vi "Correct_Disconnection_101_and_11_Point-1.vi"(4 "error IN":errorcluster, 7 "[IN] Still connected\ntracks in group":T2) -> (0 "error OUT":errorcluster, 3 "[OUT] Clusters for Re\nconstructed Tracks":T1)   [LabVIEW 2013]
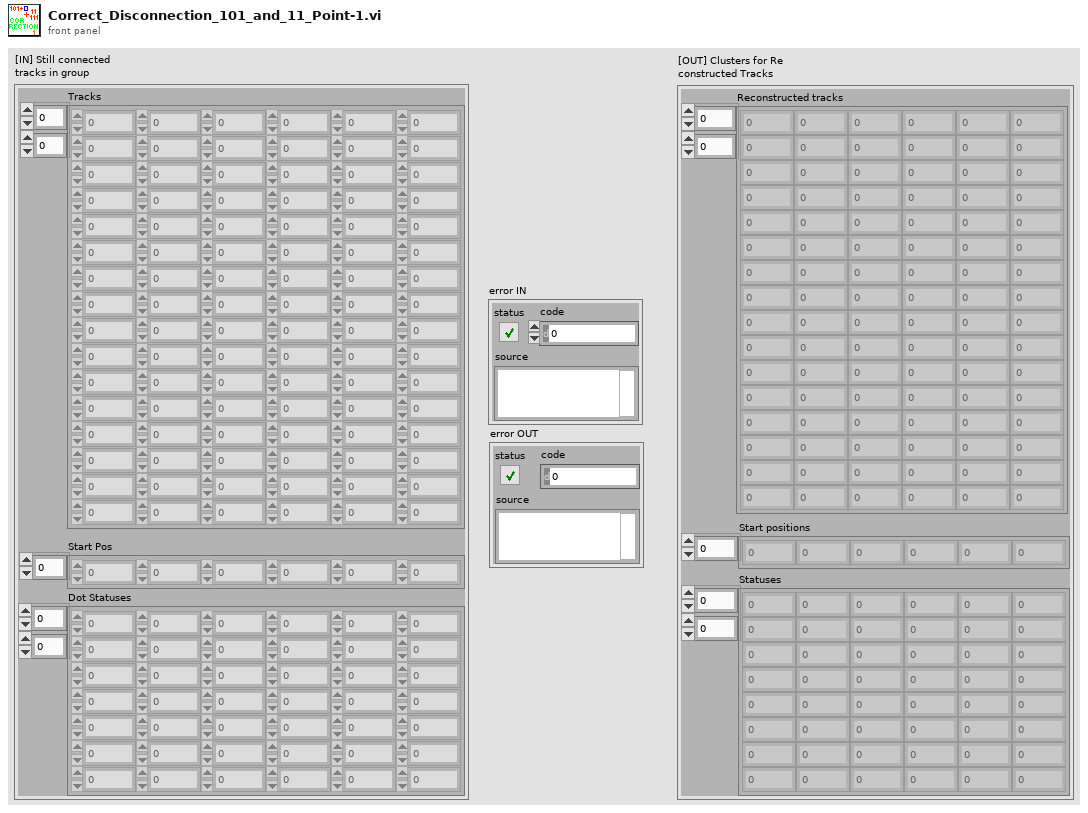
[diagram p1: front panel]
types:
  T1 = cluster{"Reconstructed tracks":dbl[][], "Start positions":i32[], "Statuses":i16[][]}
  T2 = cluster{"Tracks":dbl[][], "Start Pos":i32[], "Dot Statuses":i16[][]}
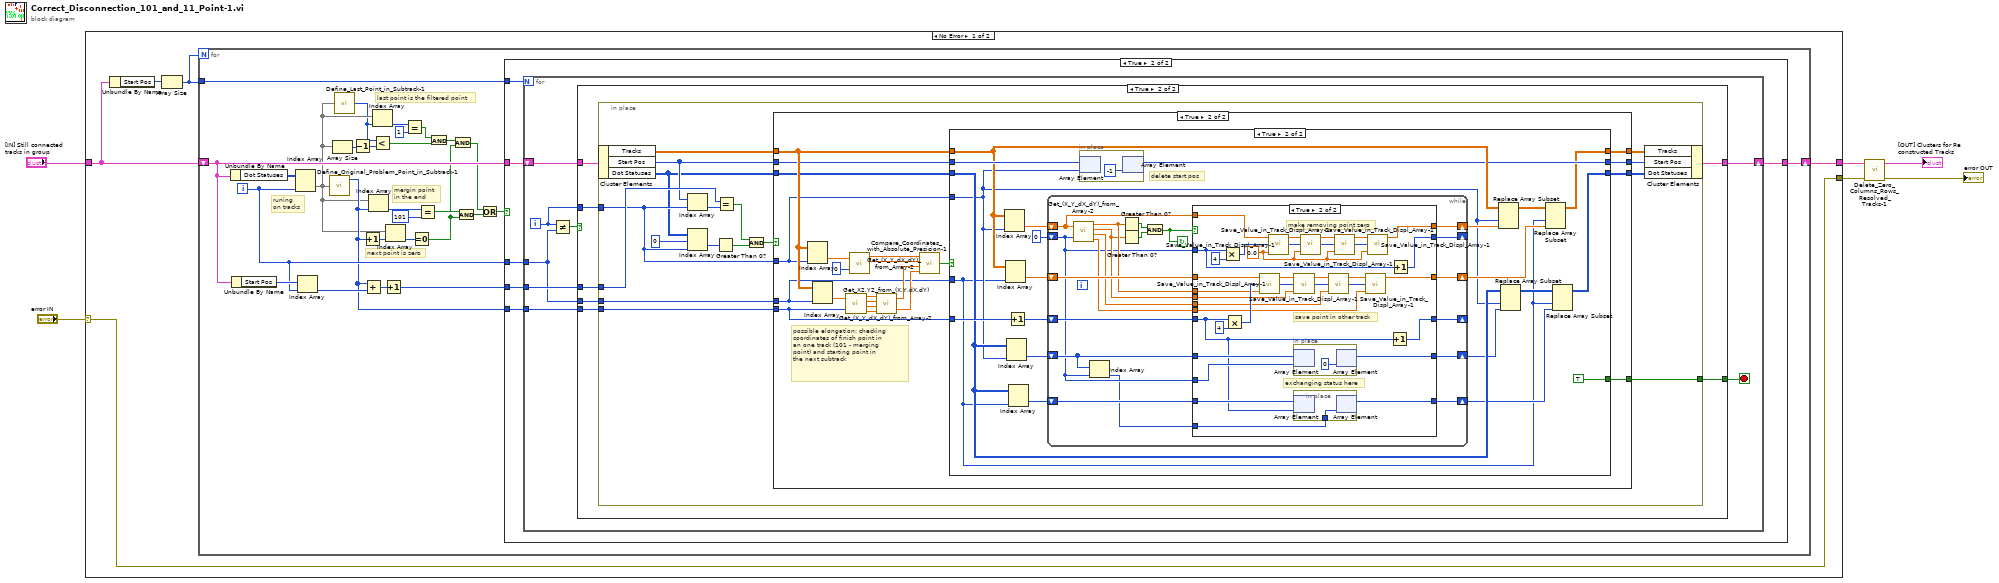
[diagram p0: block diagram]
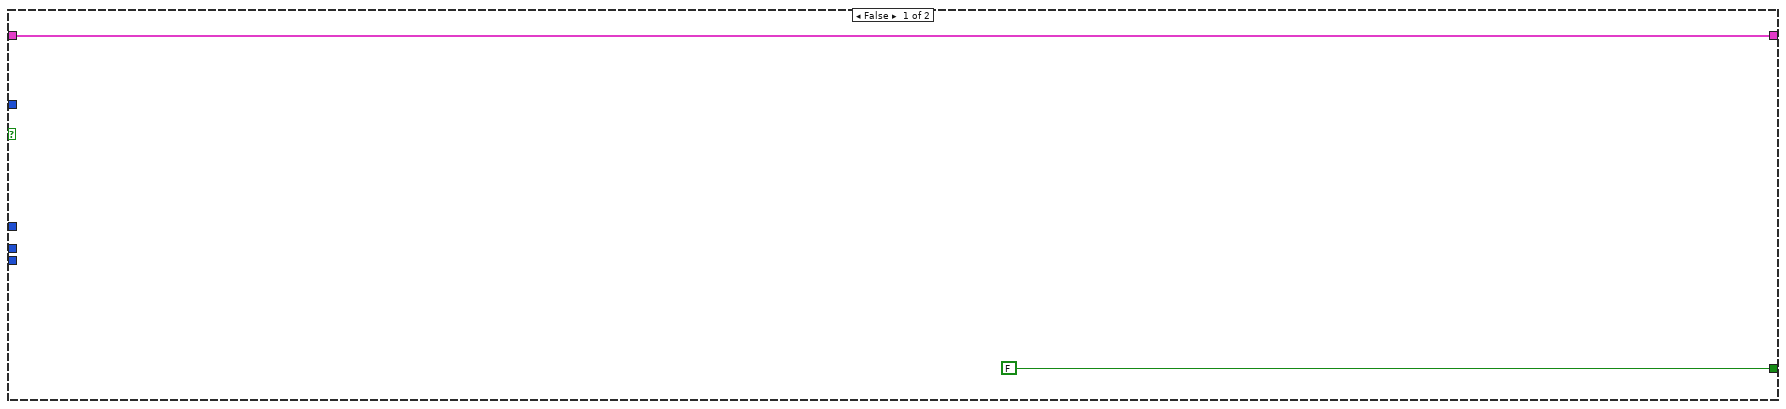
[diagram p3: hidden frame]
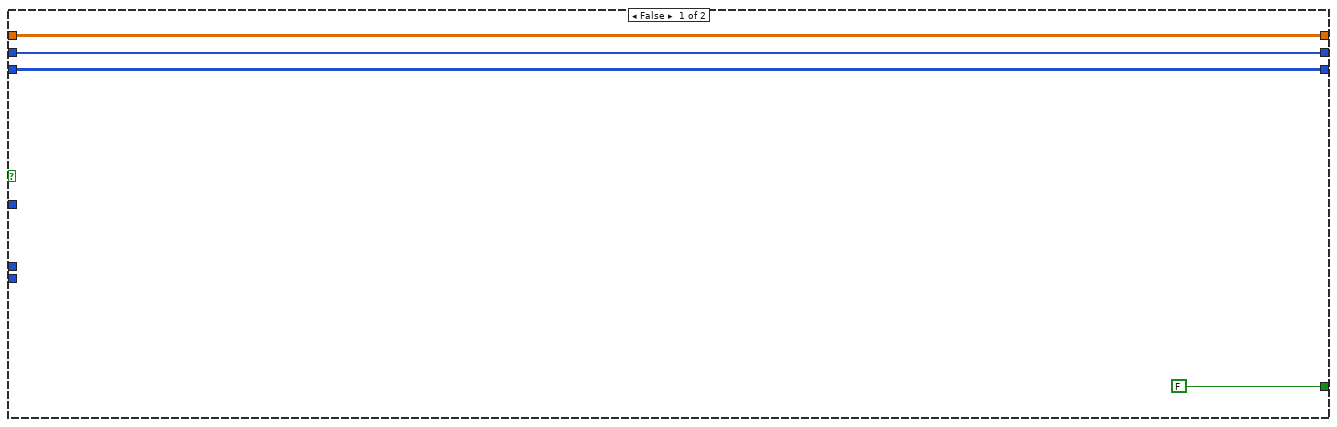
[diagram p4: hidden frame]
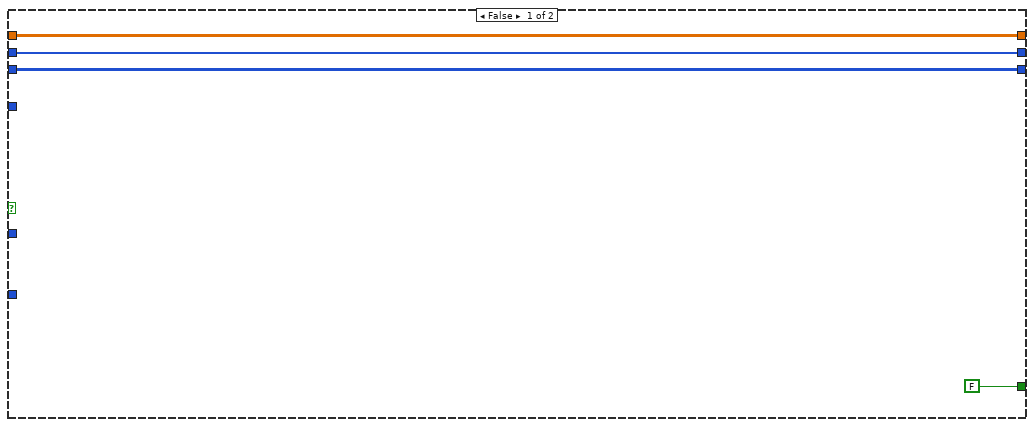
[diagram p5: hidden frame]
diagram:
  n1 = case shown="No Error" "error IN" {
    selector: "error IN" -> [w8 w197]
    tunnel: "[IN] Still connected\ntracks in group" -> [w10 w198]
    tunnel: [w8 w197] -> w3
    tunnel: [w7 w198] -> w4
    frame No Error {
      n2 = Unbundle By Name(w10) -> ("Start Pos"=w11:i32[])
      n3 = Array Size(array=w11) -> (size(s)=w9:i32)
      n4 = for {
        N: w9 -> [_]
        shift-right: [w27] -> w7
        shift-left: w10 -> [w34]
        tunnel: w9 -> [w39]
        i -> [w32]
        # "last point is the filtered point"
        # "mergin point \nin the end"
        # "runing \non tracks"
        # "next point is zero"
        n5 = Unbundle By Name(w34) -> ("Dot Statuses"=w35:i16[][])
        n6 = Unbundle By Name(w34) -> ("Start Pos"=w33:i32[])
        n7 = Index Array(array=w35, index (col)=w32) -> (element=w23:i16[])  [unwired: 1 in]
        n8 = Index Array(array=w33, index=w32) -> (element=w31:i32)
        n9 = call "Define_Original_Problem_Point_in_Subtrack-1.vi"("[IN] Statuses"=w23) -> ("[OUT] Index of Problem Point\nin Subtrack (Original)"=w28:i32)  [unwired: 3 in, 1 out]
        n10 = Array Size(array=w23) -> (size(s)=w22:i32)
        n11 = call "Define_Last_Point_in_Subtrack-1.vi"("[IN] Statuses"=w23) -> ("[OUT] Index of Problem Point\nin Subtrack (Original)"=w20:i32)  [unwired: 4 in]
        n12 = Decrement(x=w22) -> (x-1=w19:i32)
        n13 = Increment(x=w28) -> (x+1=w37:i32)
        n14 = Add(x=w28, y=w31) -> (x+y=w30:i32)
        n15 = Index Array(array=w23, index=w28) -> (element=w26:i16)
        n16 = Index Array(array=w23, index=w20) -> (element=w25:i16)
        n17 = Less?(x=w20, y=w19) -> (x < y?=w17:bool)
        n18 = Increment(x=w30) -> (x+1=w29:i32)
        n19 = Index Array(array=w23, index=w37) -> (element=w38:i16)
        n20 = Equal?(x=w25, y=i16 1) -> (x = y?=w18:bool)
        n21 = Equal To 0?(x=w38) -> (x = 0?=w15:bool)
        n22 = Equal?(x=w26, y=i16 101) -> (x = y?=w21:bool)
        n23 = And(x=w18, y=w17) -> (x .and. y?=w16:bool)
        n24 = And(x=w16, y=w15) -> (x .and. y?=w12:bool)
        n25 = And(x=w21, y=w15) -> (x .and. y?=w14:bool)
        n26 = Or(x=w12, y=w14) -> (x .or. y?=w13:bool)
        n27 = case shown="True" w13 {
          tunnel: w39 -> [_ w46]
          tunnel: w34 -> [w40 w45]
          tunnel: w32 -> [_ w44]
          tunnel: w29 -> [_ w43]
          tunnel: w28 -> [_ w42]
          tunnel: [w40 w41] -> w27
          frame False {
          }
          frame True {
            n28 = for {
              N: w46 -> [_]
              shift-right: [w48] -> w41
              shift-left: w45 -> [w53]
              tunnel: w44 -> [w50]
              tunnel: w43 -> [w51]
              tunnel: w42 -> [w49]
              i -> [w52]
              stop <- w47 stop-if-true
              n29 = Not Equal?(x=w52, y=w50) -> (x != y?=w54:bool)
              n30 = case shown="True" w54 {
                tunnel: w53 -> [w56 w63]
                tunnel: w52 -> [_ w62]
                tunnel: w51 -> [_ w61]
                tunnel: w50 -> [_ w60]
                tunnel: w49 -> [_ w59]
                tunnel: [w56 w58] -> w48
                tunnel: [FALSE w57] -> w47
                frame False {
                }
                frame True {
                  n31 = in-place {
                    in-place-border: w62 -> [w73]
                    in-place-border: w61 -> [w76]
                    in-place-border: w60 -> [w72]
                    in-place-border: w59 -> [w71]
                    in-place-border: [w65] -> w57
                    n32 = in-place-cluster #1(w63) -> ("Tracks"=w74:dbl[][], "Start Pos"=w70:i32[], "Dot Statuses"=w69:i16[][])
                    n33 = Index Array(array=w70, index=w73) -> (element=w77:i32)
                    n34 = Index Array(array=w69, index (row)=0 ("disabled index (row)"), index (col)=w73) -> (element=w78:i16)
                    n35 = Greater Than 0?(x=w78) -> (x > 0?=w64:bool)
                    n36 = Equal?(x=w76, y=w77) -> (x = y?=w79:bool)
                    n37 = And(x=w79, y=w64) -> (x .and. y?=w75:bool)
                    n38 = case shown="True" w75 {
                      tunnel: w74 -> [w84 w94]
                      tunnel: w73 -> [_ w90]
                      tunnel: w72 -> [_ w89]
                      tunnel: w71 -> [_ w91]
                      tunnel: w70 -> [w83 w93]
                      tunnel: w69 -> [w82 w92]
                      tunnel: [w83 w88] -> w68
                      tunnel: [w84 w87] -> w67
                      tunnel: [w82 w86] -> w66
                      tunnel: [FALSE w85] -> w65
                      frame False {
                      }
                      frame True {
                        # "possible elongation: checking \ncoordinates of finish point in \nan one track (101 - merging\npoint) and starting point in \nthe next subtrack"
                        n39 = Index Array(array=w94, index (col)=w90) -> (element=w106:dbl[])  [unwired: 1 in]
                        n40 = Index Array(array=w94, index (col)=w89) -> (element=w104:dbl[])  [unwired: 1 in]
                        n41 = call "Get_(X_Y_dX_dY)_from_Array-2.vi"("(X,Y,dX,dY)"=w104, "Index of Displacement"=w91) -> ("X"=w103:dbl, "Y"=w102:dbl, "dX"=w101:dbl, "dY"=w100:dbl)
                        n42 = call "Get_(X_Y_dX_dY)_from_Array-2.vi"("(X,Y,dX,dY)"=w106, "Index of Displacement"=0 ("disabled index (row)")) -> ("X"=w99:dbl, "Y"=w98:dbl)  [unwired: 2 out]
                        n43 = call "Get_X2,Y2_from_(X,Y,dX,dY).vi"("dY"=w100, "dX"=w101, "Y1"=w102, "X1"=w103) -> ("Y2 = (Y1+dY)"=w96:dbl, "X2 = (X1+dX)"=w97:dbl)
                        n44 = call "Compare_Coordinates_with_Absolute_Presicion-1.vi"("X 1"=w99, "Y 1"=w98, "X 2"=w97, "Y 2"=w96) -> ("[OUT] Same coordinates?"=w95:bool)  [unwired: 1 in]
                        n45 = case shown="True" w95 {
                          tunnel: w94 -> [w110 w124]
                          tunnel: w93 -> [w109 w132]
                          tunnel: w92 -> [w108 w120]
                          tunnel: w91 -> [_ w130]
                          tunnel: w90 -> [_ w118]
                          tunnel: w89 -> [_ w115]
                          tunnel: [w109 w114] -> w88
                          tunnel: [w110 w113] -> w87
                          tunnel: [w108 w112] -> w86
                          tunnel: [FALSE TRUE] -> w85
                          frame False {
                          }
                          frame True {
                            # "delete start pos"
                            n46 = Index Array(array=w124, index (col)=w118) -> (element=w131:dbl[])  [unwired: 1 in]
                            n47 = Index Array(array=w124, index (col)=w115) -> (element=w129:dbl[])  [unwired: 1 in]
                            n48 = Index Array(array=w120, index (col)=w118) -> (element=w126:i16[])  [unwired: 1 in]
                            n49 = Increment(x=w130) -> (x+1=w127:i32)
                            n50 = Index Array(array=w120, index (col)=w115) -> (element=w125:i16[])  [unwired: 1 in]
                            n51 = while {
                              shift-right: [w142] -> w123
                              shift-left: w131 -> [w149]
                              shift-right: [w140] -> w121
                              shift-left: w129 -> [w148]
                              shift-right: [w141] -> _
                              shift-left: 0 -> [w137]
                              shift-right: [w139] -> _
                              shift-left: w127 -> [w147]
                              shift-right: [w136] -> w119
                              shift-left: w126 -> [w138]
                              shift-right: [w133] -> w116
                              shift-left: w125 -> [w135]
                              stop <- w150 continue-if-true
                              n52 = call "Get_(X_Y_dX_dY)_from_Array-2.vi"("(X,Y,dX,dY)"=w149, "Index of Displacement"=w137) -> ("X"=w146:dbl, "Y"=w145:dbl, "dX"=w144:dbl, "dY"=w143:dbl)
                              n53 = Index Array(array=w138, index=w137) -> (element=w134:i16)
                              n54 = Greater Than 0?(x=w146) -> (x > 0?=w152:bool)
                              n55 = Greater Than 0?(x=w145) -> (x > 0?=w151:bool)
                              n56 = And(x=w152, y=w151) -> (x .and. y?=w150:bool)
                              n57 = case shown="True" w150 {
                                tunnel: w149 -> [w158 w184]
                                tunnel: w137 -> [w157 w170]
                                tunnel: w148 -> [w156 w182]
                                tunnel: w147 -> [w155 w161]
                                tunnel: w146 -> [_ w180]
                                tunnel: w145 -> [_ w177]
                                tunnel: w144 -> [_ w174]
                                tunnel: w143 -> [_ w171]
                                tunnel: [w158 w169] -> w142
                                tunnel: [w157 w168] -> w141
                                tunnel: [w156 w167] -> w140
                                tunnel: [w155 w166] -> w139
                                tunnel: w138 -> [w154 w165]
                                tunnel: w137 -> [_ w164]
                                tunnel: [w154 w163] -> w136
                                tunnel: w135 -> [w153 w162]
                                tunnel: w134 -> [_ w160]
                                tunnel: [w153 w159] -> w133
                                frame False {
                                }
                                frame True {
                                w193 = 0.0 ("[IN] Value")
                                # "exchanging status here"
                                # "make removing point zero"
                                # "save point in other track"
                                n58 = Multiply(x=w170, y=4) -> (x*y=w185:i32)
                                n59 = Multiply(x=w161, y=4) -> (x*y=w181:i32)
                                n60 = call "Save_Value_in_Track_Displ_Array-1.vi"("[IN] Value"=w180, "[IN] Index"=w181, "[IN] Empty tracks\nfor points saving"=w182) -> ("[OUT] Index ++"=w178:i32, "[OUT Track with saved value"=w179:dbl[])  [unwired: 1 in]
                                n61 = call "Save_Value_in_Track_Displ_Array-1.vi"("[IN] Value"=w193, "[IN] Index"=w185, "[IN] Empty tracks\nfor points saving"=w184) -> ("[OUT] Index ++"=w188:i32, "[OUT Track with saved value"=w187:dbl[])  [unwired: 1 in]
                                n62 = call "Save_Value_in_Track_Displ_Array-1.vi"("[IN] Value"=w177, "[IN] Index"=w178, "[IN] Empty tracks\nfor points saving"=w179) -> ("[OUT] Index ++"=w175:i32, "[OUT Track with saved value"=w176:dbl[])  [unwired: 1 in]
                                n63 = in-place {
                                n64 = in-place-array #2(w165, w164) -> ()  [unwired: 1 out]
                                n65 = in-place-array #2(i16 0 ("element")) -> (w163:i16[])  [unwired: 1 out]
                                }
                                n66 = in-place {
                                in-place-border: w160 -> [w194]
                                n67 = in-place-array #3(w162, w161) -> ()  [unwired: 1 out]
                                n68 = in-place-array #3(w194) -> (w159:i16[])  [unwired: 1 out]
                                }
                                n69 = call "Save_Value_in_Track_Displ_Array-1.vi"("[IN] Value"=w193, "[IN] Index"=w188, "[IN] Empty tracks\nfor points saving"=w187) -> ("[OUT] Index ++"=w190:i32, "[OUT Track with saved value"=w189:dbl[])  [unwired: 1 in]
                                n70 = call "Save_Value_in_Track_Displ_Array-1.vi"("[IN] Value"=w174, "[IN] Index"=w175, "[IN] Empty tracks\nfor points saving"=w176) -> ("[OUT] Index ++"=w172:i32, "[OUT Track with saved value"=w173:dbl[])  [unwired: 1 in]
                                n71 = call "Save_Value_in_Track_Displ_Array-1.vi"("[IN] Value"=w193, "[IN] Index"=w190, "[IN] Empty tracks\nfor points saving"=w189) -> ("[OUT] Index ++"=w192:i32, "[OUT Track with saved value"=w191:dbl[])  [unwired: 1 in]
                                n72 = call "Save_Value_in_Track_Displ_Array-1.vi"("[IN] Value"=w171, "[IN] Index"=w172, "[IN] Empty tracks\nfor points saving"=w173) -> ("[OUT Track with saved value"=w167:dbl[])  [unwired: 1 in, 1 out]
                                n73 = call "Save_Value_in_Track_Displ_Array-1.vi"("[IN] Value"=w193, "[IN] Index"=w192, "[IN] Empty tracks\nfor points saving"=w191) -> ("[OUT Track with saved value"=w169:dbl[])  [unwired: 1 in, 1 out]
                                n74 = Increment(x=w161) -> (x+1=w166:i32)
                                n75 = Increment(x=w170) -> (x+1=w168:i32)
                                }
                              }
                            }
                            n76 = in-place {
                              n77 = in-place-array #4(w132, w118) -> ()  [unwired: 1 out]
                              n78 = in-place-array #4(-1) -> (w114:i32[])  [unwired: 1 out]
                            }
                            n79 = Replace Array Subset(array=w124, new element=w123, index (col)=w118) -> (w122:dbl[][])  [unwired: 1 in]
                            n80 = Replace Array Subset(array=w120, new element=w119, index (col)=w118) -> (w117:i16[][])  [unwired: 1 in]
                            n81 = Replace Array Subset(array=w122, new element=w121, index (col)=w115) -> (w113:dbl[][])  [unwired: 1 in]
                            n82 = Replace Array Subset(array=w117, new element=w116, index (col)=w115) -> (w112:i16[][])  [unwired: 1 in]
                          }
                        }
                      }
                    }
                    n83 = in-place-cluster #1("Tracks"=w67, "Start Pos"=w68, "Dot Statuses"=w66) -> (w58:T2)
                  }
                }
              }
            }
          }
        }
      }
    }
    frame Error {
    }
  }
  n84 = call "Delete_Zero_Columns_Rows_Resolved_Tracks-1.vi"("error IN"=w3, "[IN] Clusters for Re\nconstructed Tracks"=w4) -> ("error OUT"=→"error OUT":errorcluster, "[OUT] Clusters for Re\nconstructed Tracks"=→"[OUT] Clusters for Re\nconstructed Tracks":T1)  [unwired: 4 in]
